vi "Test Delete Node.vi"(8 "error in (no error)":errorcluster) -> (0 "error out":errorcluster)   [LabVIEW 2017, in "Unit Tests.lvlib"]
uses:
  Unit Tests.lvlib
  source/Browser Core/Node Classes/Generic Node/Generic Node.lvclass/Generic Node.ctl
  source/Browser Core/Server Classes/Base Tree/Base Tree.lvclass
  <vilib>/addons/_JKI Toolkits/Caraya/classes/Test/Test.lvclass
  <vilib>/addons/_JKI Toolkits/Caraya/classes/Assert/Assert.lvclass
  source/Browser Core/Node Classes/Generic Node/Generic Node.lvclass
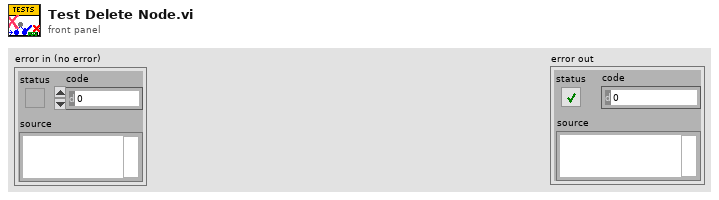
[diagram p1: front panel]
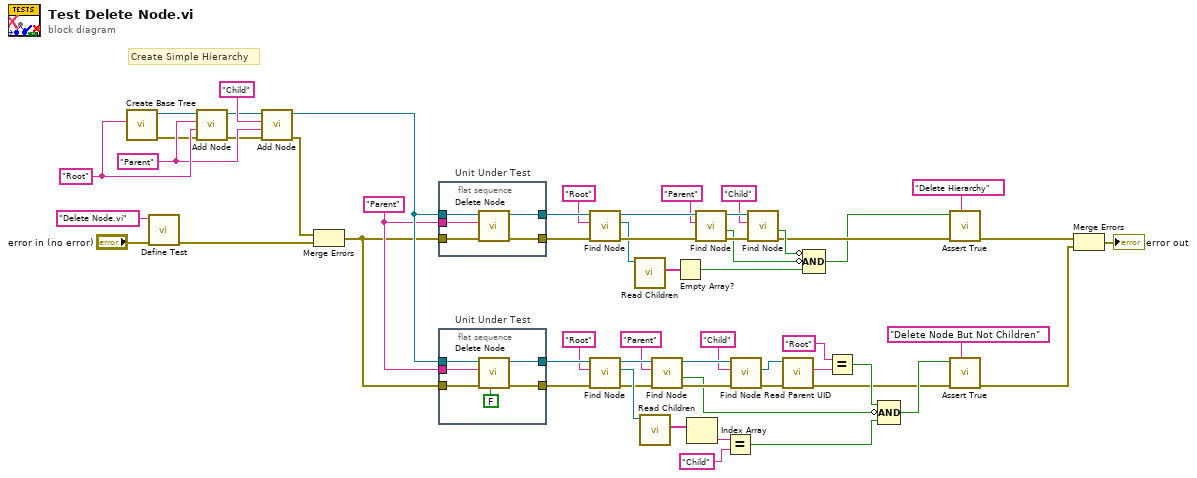
[diagram p0: block diagram]
diagram:
  w41 = "Parent" ("UID")
  w49 = "Parent" ("UID")
  w50 = "Root" ("Root UID")
  # "Create Simple Hierarchy"
  n1 = call "Create Base Tree.vi"("Root UID"=w50) -> ("error out"=w46:errorcluster, "Base Tree out"=w51:refnum<class "Base Tree.lvclass">)  [unwired: 9 in]
  n2 = call <vilib>:"Define Test.vi"("error in (no error)"="error in (no error)", "Label (VI Title)"="Delete Node.vi") -> ("error out"=w44:errorcluster)  [unwired: 9 in]
  n3 = call-dynamic "Add Node.vi"("error in (no error)"=w46, "Parent"=w50, "UID"=w49, "Base Tree in"=w51) -> ("error out"=w45:errorcluster, "Base Tree out"=w47:refnum<class "Base Tree.lvclass">)  [unwired: 6 in]
  n4 = call-dynamic "Add Node.vi"("error in (no error)"=w45, "Parent"=w49, "UID"="Child", "Base Tree in"=w47) -> ("error out"=w43:errorcluster, "Base Tree out"=w42:refnum<class "Base Tree.lvclass">)  [unwired: 6 in]
  n5 = Merge Errors(w43, w44) -> (w40:errorcluster)
  n6 = flat-sequence "Unit Under Test" {
    tunnel: w40 -> [w62]
    tunnel: w42 -> [w61]
    tunnel: w41 -> [w60]
    tunnel: [w59] -> w39
    tunnel: [w58] -> w38
    frame #0 {
      n7 = call-dynamic "Delete Node.vi"("error in (no error)"=w62, "UID"=w60, "Base Tree in"=w61) -> ("error out"=w58:errorcluster, "Base Tree out"=w59:refnum<class "Base Tree.lvclass">)  [unwired: 7 in]
    }
  }
  n8 = flat-sequence "Unit Under Test" {
    tunnel: w40 -> [w68]
    tunnel: w42 -> [w67]
    tunnel: w41 -> [w66]
    tunnel: [w64] -> w22
    tunnel: [w63] -> w21
    frame #0 {
      n9 = call-dynamic "Delete Node.vi"("Remove Children? (T)"=FALSE, "error in (no error)"=w68, "UID"=w66, "Base Tree in"=w67) -> ("error out"=w63:errorcluster, "Base Tree out"=w64:refnum<class "Base Tree.lvclass">)  [unwired: 6 in]
    }
  }
  n10 = call-dynamic "Find Node.vi"("error in (no error)"=w38, "UID"="Root", "Base Tree in"=w39) -> ("error out"=w37:errorcluster, "Node"=w30:refnum<class "Generic Node.lvclass">, "Base Tree out"=w36:refnum<class "Base Tree.lvclass">)  [unwired: 5 in, 1 out]
  n11 = call-dynamic "Find Node.vi"("error in (no error)"=w21, "UID"="Root", "Base Tree in"=w22) -> ("error out"=w14:errorcluster, "Node"=w19:refnum<class "Generic Node.lvclass">, "Base Tree out"=w15:refnum<class "Base Tree.lvclass">)  [unwired: 5 in, 1 out]
  n12 = call "Read Children.vi"("Generic Node in"=w30) -> ("Children"=w27:string[])  [unwired: 8 in, 2 out]
  n13 = call "Read Children.vi"("Generic Node in"=w19) -> ("Children"=w18:string[])  [unwired: 8 in, 2 out]
  n14 = call-dynamic "Find Node.vi"("error in (no error)"=w14, "UID"="Parent", "Base Tree in"=w15) -> ("error out"=w12:errorcluster, "Found?"=w5:bool, "Base Tree out"=w11:refnum<class "Base Tree.lvclass">)  [unwired: 5 in, 1 out]
  n15 = Empty Array?(array=w27) -> (empty?=w26:bool)
  n16 = Index Array(array=w18) -> (element=w17:string)  [unwired: 1 in]
  n17 = call-dynamic "Find Node.vi"("error in (no error)"=w37, "UID"="Parent", "Base Tree in"=w36) -> ("error out"=w35:errorcluster, "Found?"=w28:bool, "Base Tree out"=w34:refnum<class "Base Tree.lvclass">)  [unwired: 5 in, 1 out]
  n18 = Equal?(x=w17, y="Child" ("UID")) -> (x = y?=w3:bool)
  n19 = call-dynamic "Find Node.vi"("error in (no error)"=w12, "UID"="Child", "Base Tree in"=w11) -> ("error out"=w8:errorcluster, "Node"=w9:refnum<class "Generic Node.lvclass">)  [unwired: 5 in, 2 out]
  n20 = call-dynamic "Find Node.vi"("error in (no error)"=w35, "UID"="Child", "Base Tree in"=w34) -> ("error out"=w25:errorcluster, "Found?"=w29:bool)  [unwired: 5 in, 2 out]
  n21 = call "Read Parent UID.vi"("error in (no error)"=w8, "Generic Node in"=w9) -> ("error out"=w1:errorcluster, "Parent UID"=w7:string)  [unwired: 7 in, 1 out]
  n22 = Compound Arithmetic op=AND(invert w29, invert w28, w26) -> (w24:bool)
  n23 = Equal?(x="Root" ("UID"), y=w7) -> (x = y?=w4:bool)
  n24 = Compound Arithmetic op=AND(w4, invert w5, w3) -> (w2:bool)
  n25 = call <vilib>:"Assert True.vi"("Label"="Delete Hierarchy", "error in (no error)"=w25, "True?"=w24) -> ("error out"=w54:errorcluster)  [unwired: 8 in]
  n26 = call <vilib>:"Assert True.vi"("Label"="Delete Node But Not Children", "error in (no error)"=w1, "True?"=w2) -> ("error out"=w53:errorcluster)  [unwired: 8 in]
  n27 = Merge Errors(w54, w53) -> (→"error out":errorcluster)
